vi "if_T.vi"() -> ()   [LabVIEW 2019]
panel:
  out "x-y":u32
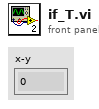
[diagram p1: front panel]
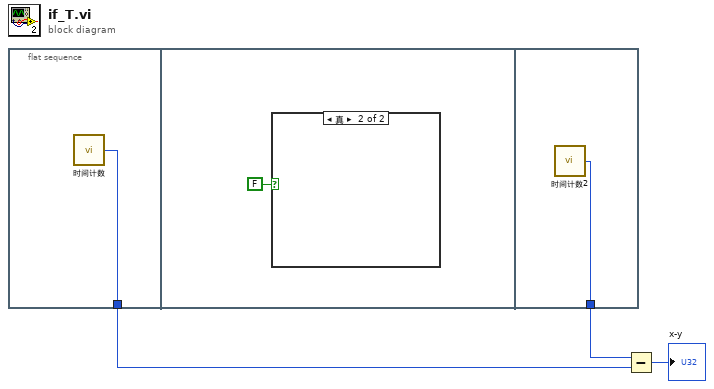
[diagram p0: block diagram]
diagram:
  n1 = flat-sequence {
    tunnel: [w4] -> w2
    tunnel: [w6] -> w3
    frame #0 {
      n2 = call "时间计数"() -> ("Tick Count(Ticks)"=w4:u32)
    }
    frame #1 {
      n3 = case shown="真" FALSE {
        frame False {
        }
        frame True {
        }
      }
    }
    frame #2 {
      n4 = call "时间计数2"() -> ("Tick Count(Ticks)"=w6:u32)
    }
  }
  n5 = Subtract(x=w3, y=w2) -> (x-y=→"x-y":u32)
